vi "Action - TDMS Defragment.vi"(8 "error in (no error)":errorcluster, 11 "file path":path) -> (0 "error out":errorcluster)   [LabVIEW 2021, in "XNET-CAN-Signal-Logger.lvlib"]
uses:
  XNET-CAN-Signal-Logger.lvlib
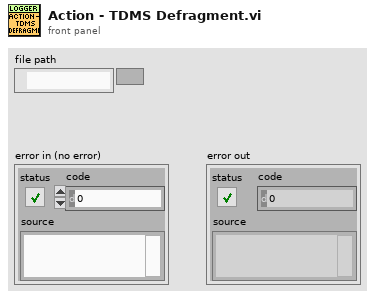
[diagram p1: front panel]
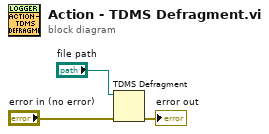
[diagram p0: block diagram]
diagram:
  n1 = TDMS Defragment(4:"error in (no error)", 7:"file path") -> (0:→"error out":errorcluster)
